vi "sem_post.vi"(8 "error in (no error)":errorcluster, 11 "sempahore ptr in":u64) -> (0 "error out":errorcluster, 3 "semaphore ptr out":u64)   [LabVIEW 2013, in "POSIX Threads.lvlib" / "POSIX Thread Object.lvclass"]
uses:
  POSIX Thread Object.lvclass
  Controls/pthread functions.ctl
  <vilib>/NI/NI Linux RT Errno/Linux Errno.lvlib
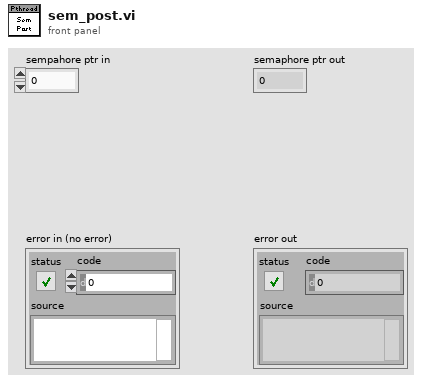
[diagram p1: front panel]
types:
  T1 = typedef "POSIX Threads.lvlib/POSIX Thread Object.lvclass/pthread functions.ctl" = enum16{"unspecified", "pthread_condattr_init", "pthread_condattr_destroy", "pthread_condattr_getclock", "pthread_condattr_setclock", "pthread_condattr_getpshared", "pthread_condattr_setpshared", "pthread_cond_init", "pthread_cond_destroy", "pthread_cond_broadcast", "pthread_cond_signal", "pthread_cond_timedwait", "pthread_cond_wait", "pthread_mutexattr_init", "pthread_mutexattr_destroy", "pthread_mutexattr_getprioceiling", "pthread_mutexattr_setprioceiling", "pthread_mutexattr_getprotocol", "pthread_mutexattr_setprotocol", "pthread_mutexattr_getpshared", "pthread_mutexattr_setpshared", "pthread_mutexattr_gettype", "pthread_mutexattr_settype", "pthread_mutex_init", "pthread_mutex_destroy", "pthread_mutex_getprioceiling", "pthread_mutex_setprioceiling", "pthread_mutex_lock", "pthread_mutex_timedlock", "pthread_mutex_trylock", "pthread_mutex_unlock", "sem_destroy", "sem_getvalue", "sem_init", "sem_post", "sem_timedwait", "sem_trywait", "sem_wait", "barrier_init", "barrier_destroy", "barrier_wait", "barrierattr_init", "barrierattr_destroy", "barrierattr_getpshared", "barrierattr_setpshared"}
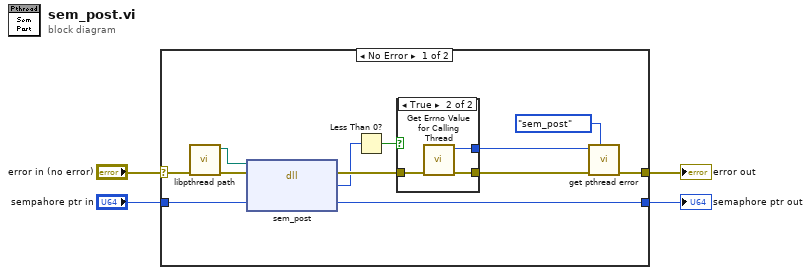
[diagram p0: block diagram]
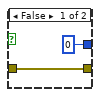
[diagram p2: hidden frame]
diagram:
  n1 = case shown="No Error" "error in (no error)" {
    selector: "error in (no error)" -> [w16 w23]
    tunnel: "sempahore ptr in" -> [w15 w22]
    tunnel: [w14 w23] -> w2
    tunnel: [w13 w22] -> w1
    frame No Error {
      n2 = call "libpthread path.vi"("error in (no error)"=w16) -> ("error out"=w11:errorcluster, "path to libpthread"=w12:path)  [unwired: 9 in]
      n3 = dll-call lib="?" fn="sem_post"(path in=w12, error in=w11, "sem"=w15) -> (error out=w8:errorcluster, "errno"=w7:i32, "sem"=w13:u64)  [unwired: 1 in, 1 out]
      n4 = Less Than 0?(x=w7) -> (x < 0?=w9:bool)
      n5 = case shown="True" w9 {
        tunnel: w8 -> [w18 w21]
        tunnel: [w18 w20] -> w6
        tunnel: [0 ("errno") w19] -> w5
        frame False {
        }
        frame True {
          n6 = call <vilib>:"Get Errno Value for Calling Thread.vi"("error in (no error)"=w21) -> ("error out"=w20:errorcluster, "errno"=w19:i32)  [unwired: 9 in]
        }
      }
      n7 = call "get pthread error.vi"("function"=pthread_functions."sem_post", "error in (no error)"=w6, "errno"=w5) -> ("error out"=w14:errorcluster)  [unwired: 8 in]
    }
    frame Error {
    }
  }
  "error out" <- w2
  "semaphore ptr out" <- w1
